vi "ARM_MOVE.vi"(10 "argv":string[](array[string]), 11 "args":u8) -> ()   [LabVIEW 2014]
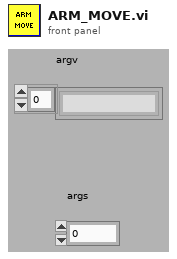
[diagram p1: front panel]
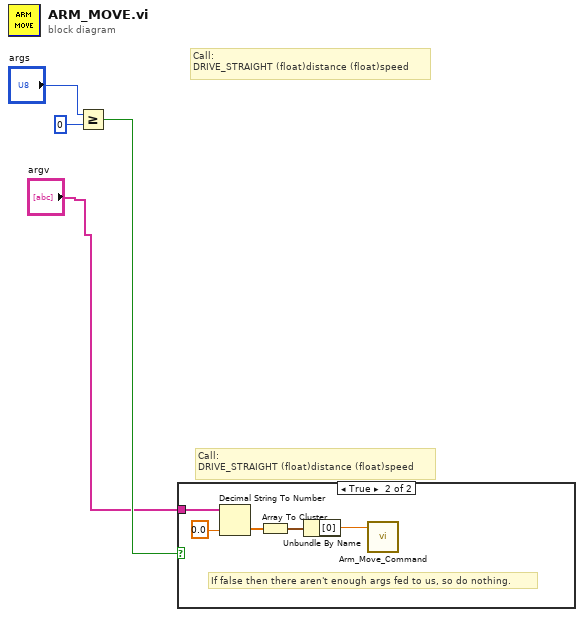
[diagram p0: block diagram]
diagram:
  # "Call:\nDRIVE_STRAIGHT (float)distance (float)speed"
  # "Call:\nDRIVE_STRAIGHT (float)distance (float)speed"
  n1 = Greater Or Equal?(x="args", y=u8 0) -> (x >= y?=w4:bool)
  n2 = case shown="True" w4 {
    tunnel: "argv" -> [_ w9]
    frame False {
    }
    frame True {
      # "If false then there aren't enough args fed to us, so do nothing."
      n3 = Decimal String To Number(string=w9, default (0L)=0.0 ("default (0 I32)")) -> (number=w7:dbl[])  [unwired: 2 out]
      n4 = Array To Cluster(array=w7) -> (cluster=w6:cluster{"[0]":dbl, "[1]":dbl})
      n5 = Unbundle By Name(w6) -> ("[0]"=w5:dbl)
      n6 = call "Arm_Move_Command.vi"("Argument"=w5) -> ()  [unwired: 11 in]
    }
  }
